vi "Actor Core.vi"(8 "error in":errorcluster, 11 "Measure Object in":refnum<class "Ruby Spectra.lvclass">) -> (0 "error out":errorcluster, 3 "Actor out":refnum<class "Actor.lvclass">)   [LabVIEW 2016, in "Ruby Spectra.lvclass"]
doc: "(<B>Filename</B>: Actor Framework.lvlib:Actor.lvclass:Actor Core.vi)\n\nReceives messages to the actor, reacts to them, and initiates any error handling that may shut the actor down.\n\nDescendant classes may override this VI to append parallel tasks for the actor to complete while it handles messages. Overrides use the Call Parent Method node."
uses:
  Ruby Spectra.lvclass
  C:/github/LabActor/Template Module/Template Module.lvclass
  C:/github/LabActor/Recorders/Spectrometer/Spectrometer.lvclass
  C:/Program Files/National Instruments/LabVIEW 2016/vi.lib/ActorFramework/Actor/Actor.lvclass
  <vilib>/ActorFramework/Actor/Actor.lvclass
  NHMFL_Core/Libraries/Instruments/Ocean Optics/Ocean Optics Driver/Ocean optics configuration.ctl
  NHMFL_Core/Libraries/Utilities/Fit/Multi-peak Parameters.ctl
  NHMFL_Core/Libraries/Utilities/Fit/Peak Parameters.ctl
  Ruby Spectra.lvclass/Ruby Spectra.ctl
  Template Module/Template Module.lvclass/Template Module.ctl
  Spectrometer/Spectrometer.lvclass/Spectrometer.ctl
  <vilib>/ActorFramework/Actor/Actor.lvclass/Actor.ctl
  <vilib>/ActorFramework/Message Enqueuer/Message Enqueuer.lvclass/Message Enqueuer.ctl
  Micron Optics Recorder Messages/Plot Spectrum Msg/Plot Spectrum Msg.lvclass/Plot Spectrum Msg.ctl
  Template Module/Read stop event.vi
  Spectrometer/Write Spectrum Graph ref.vi
  <vilib>/ActorFramework/Message Enqueuer/Init from Existing Queue.vi
  <vilib>/ActorFramework/Message Enqueuer/Enqueue.vi
  Micron Optics Recorder Messages/Plot Spectrum Msg/Plot Spectrum Msg.lvclass
  C:/Program Files/National Instruments/LabVIEW 2016/vi.lib/ActorFramework/Message/Message.lvclass
  <vilib>/ActorFramework/Message Priority Queue/Priority Enqueue.vi
  Spectrometer/Spectrometer.lvclass
  <vilib>/ActorFramework/Message Enqueuer/Message Enqueuer.lvclass
panel:
  out "Pressure":dbl format="%#_4pPa"
  in  "Refresh  specrum":bool
  in  "Save spectrum":bool
  out "Spectral Waveform":T1(graph)
  in  "Configuration":T2={"Integration time"=0.5, "Fit parameters"={"Function"=enum."Lorentz", "Window width"=0.5, "Initial guess"={"Amplitude"=1000.0, "Center"=694.3, "Width"=0.4}}, "Fit"=FALSE, "Auto-update params"=TRUE, "Save spectra"=TRUE, "Reference wavelengh"=694.3, "Background"=path ""} {"Reference wavelengh" format="%#_gnm"; "Fit parameters"."Initial guess"."Width" format="%#_gnm"; "Fit parameters"."Initial guess"."Center" format="%#_gnm"; "Fit parameters"."Window width" format="%#_6gnm"; "Integration time" format="%#_6ps"}
  out "Name":string
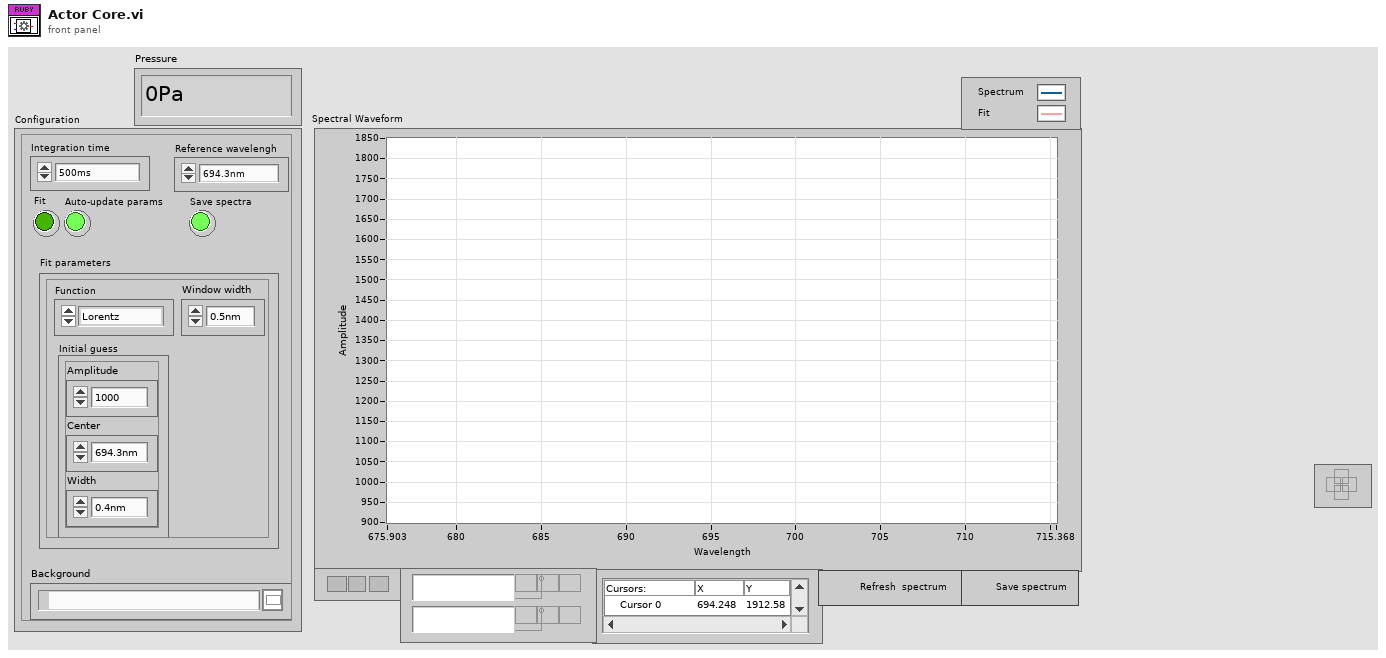
[diagram p1: front panel]
types:
  T1 = cluster{"Wavelength (nm)":dbl[], "Spectrum by Pixel Number":dbl[]}[]
  T2 = typedef "Ruby Spectra.lvclass/Ocean optics configuration.ctl" = cluster{"Integration time":dbl, "Fit parameters":T3, "Fit":bool, "Auto-update params":bool, "Save spectra":bool, "Reference wavelengh":dbl, "Background":path}
  T3 = typedef "Multi-peak Parameters.ctl" = cluster{"Function":enum16{"Gauss", "Lorentz"}, "Window width":dbl, "Initial guess":T4}
  T4 = typedef "Peak Parameters.ctl" = cluster{"Amplitude":dbl, "Center":dbl, "Width":dbl}
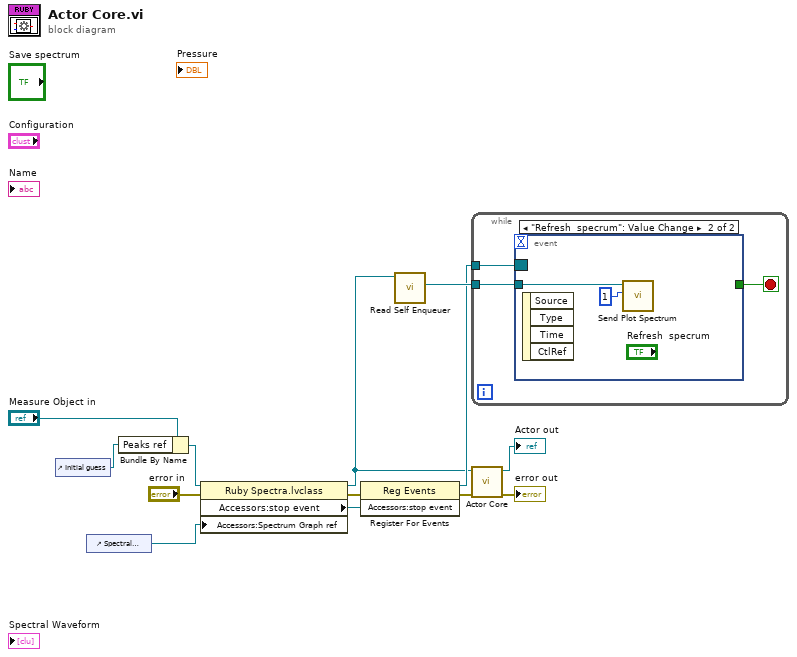
[diagram p0: block diagram]
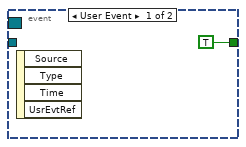
[diagram p2: hidden frame]
diagram:
  n1 = control-ref of="Initial guess"() -> (w1:refnum<vi>)
  n2 = control-ref of="Spectral Waveform"() -> (w5:refnum<vi>)
  n3 = Bundle By Name(cluster="Measure Object in", "Peaks ref"=w1) -> (w2:refnum<class "Ruby Spectra.lvclass">)
  n4 = property class="Ruby Spectra.lvclass"(reference=w2, error in="error in", "Accessors:Spectrum Graph ref"=w5) -> (reference out=w4:refnum<class "Ruby Spectra.lvclass">, error out=w8:errorcluster, "Accessors:stop event"=w7:refnum<user-event>)
  n5 = register-events(error in=w8, w7) -> (reference out=w9:refnum<event-registration>, error out=w3:errorcluster)  [unwired: 1 in]
  n6 = call <vilib>:"Read Self Enqueuer.vi"("Actor"=w4) -> ("Self Enqueuer"=w10:refnum<class "Message Enqueuer.lvclass">)  [unwired: 10 in]
  n7 = while {
    tunnel: w9 -> [w16]
    tunnel: w10 -> [w14]
    stop <- w15 stop-if-true
    n8 = event shown="[1] \"Refresh  specrum\": Value Change" {
      selector: w16 -> [_ _]
      dyn-events: _ -> [_ _]
      timeout: _ -> [_ _]
      tunnel: [TRUE _] -> w15
      tunnel: w14 -> [_ w19]
      event User Event {
        n9 = event-data() -> ()  [unwired: 1 in, 4 out]
      }
      event "Refresh  specrum": Value Change {
        n10 = event-data() -> ()  [unwired: 1 in, 4 out]
        n11 = call "Send Plot Spectrum.vi"("Channel"=u8 1, "Message Enqueuer"=w19) -> ()  [unwired: 8 in, 2 out]
      }
    }
  }
  n12 = call-parent "Actor Core.vi"("error in"=w3, "Measure Object in"=w4) -> ("error out"=→"error out":errorcluster, "Actor out"=→"Actor out":refnum<class "Actor.lvclass">)  [unwired: 8 in]
